vi "Update Gas desk files.vi"() -> ()   [LabVIEW 2011]
uses:
  Controls/File_Selector_Type.ctl
panel:
  out "Current file":path
  in  "Previous Choice":path
  in  "Search String":string
  in  "At Dialog Prompt Post Process":T1
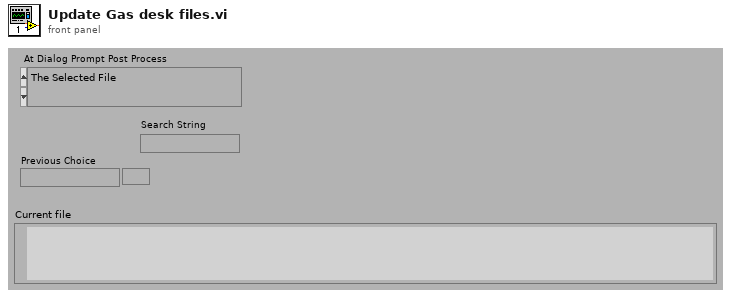
[diagram p1: front panel]
types:
  T1 = typedef "File_Selector_Type.ctl" = enum16{"The Selected File", "The Selected Folder", "Files containing the search string in the selected folder", "All files listed in selected file"}
  T2 = enum16{"To Traverse Coordinates", "To User Coordinates"}
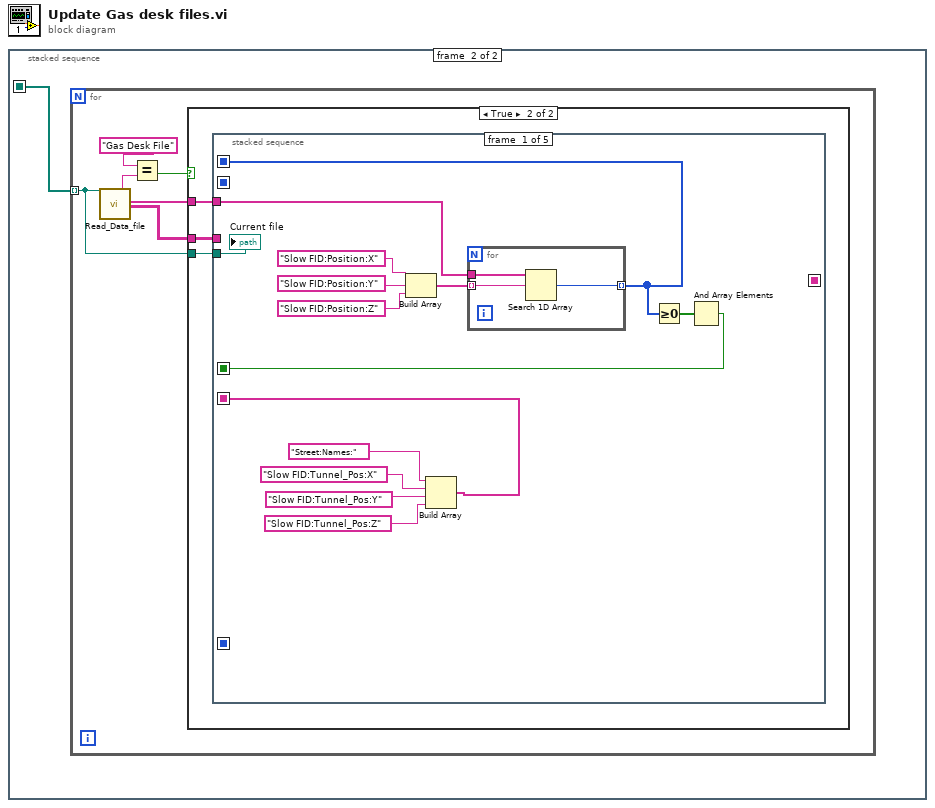
[diagram p0: block diagram]
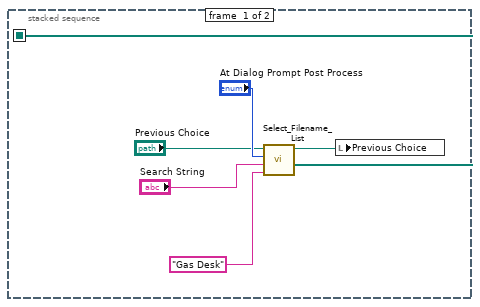
[diagram p2: hidden frame]
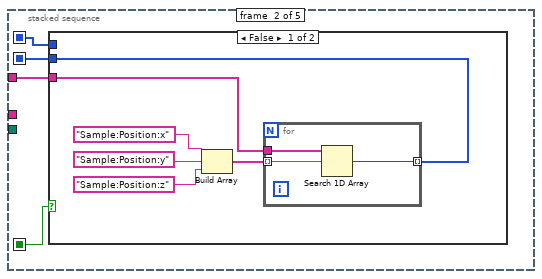
[diagram p4: hidden frame]
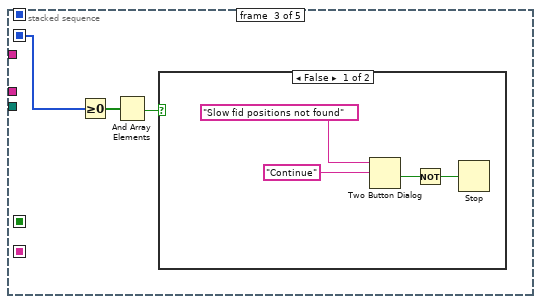
[diagram p6: hidden frame]
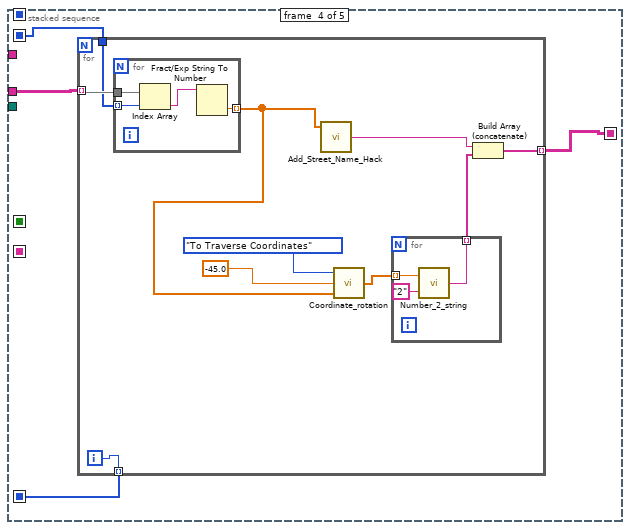
[diagram p8: hidden frame]
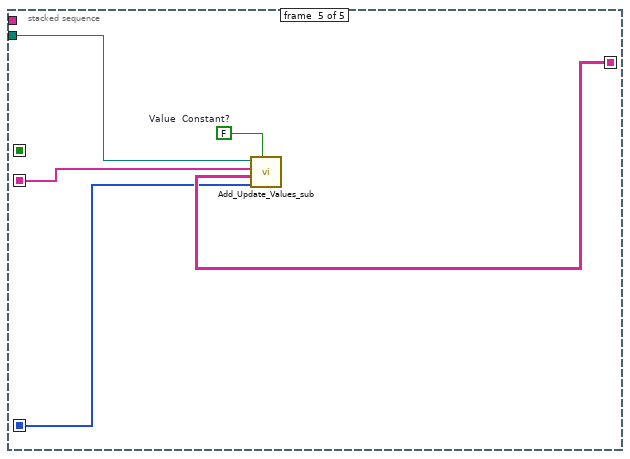
[diagram p9: hidden frame]
diagram:
  n1 = stacked-sequence {
    seq-local: [w1 _] -> [_ w7]
    frame #0 {
      n2 = call "Select_Filename_List.vi"("File Type"="Gas Desk", "Search String"="Search String", "At Dialog Prompt Post Process"="At Dialog Prompt Post Process", "Previous Choice"="Previous Choice") -> ("Selected files"=w1:path[], "Choosen path"=w4:path)  [unwired: 2 in, 1 out]
      n3 = local write "Previous Choice"(w4) -> ()
    }
    frame #1 {
      n4 = for {
        tunnel: w7 -> [w8] mode=indexing
        n5 = call "Read_Data_file.vi"("Results file"=w8) -> ("Filetype"=w13:string, "Ch names Out"=w10:string[], "Channel Values Out"=w9:string[][])  [unwired: 9 in, 7 out]
        n6 = Equal?(x="Gas Desk File", y=w13) -> (x = y?=w11:bool)
        n7 = case shown="True" w11 {
          tunnel: w10 -> [_ w16]
          tunnel: w9 -> [_ w15]
          tunnel: w8 -> [_ w14]
          frame False {
          }
          frame True {
            n8 = stacked-sequence {
              seq-local: [w20 _ _ _ _] -> [_ w34 _ _ _]
              seq-local: [w21 _ _ _ _] -> [_ _ _ _ w79]
              seq-local: [_ _ _ w57 _] -> [_ _ _ _ w78]
              seq-local: [_ _ _ w56 _] -> [_ _ _ _ w77]
              seq-local: [w18 _ _ _ _] -> [_ w36 _ _ _]
              seq-local: [_ w35 _ _ _] -> [_ _ w49 w55 _]
              tunnel: w16 -> [w26 w37 _ _ _]
              tunnel: w15 -> [_ _ _ w58 _]
              tunnel: w14 -> [w17 _ _ _ w80]
              frame #0 {
                n9 = Build Array("Slow FID:Position:X", "Slow FID:Position:Y", "Slow FID:Position:Z") -> (w27:string[])
                n10 = Build Array("Street:Names:", "Slow FID:Tunnel_Pos:X", "Slow FID:Tunnel_Pos:Y", "Slow FID:Tunnel_Pos:Z") -> (w21:string[])
                n11 = for {
                  tunnel: w27 -> [w33] mode=indexing
                  tunnel: w26 -> [w32]
                  tunnel: [w31] -> w20 mode=indexing
                  n12 = Search 1D Array(1D array=w32, element=w33) -> (index of element=w31:i32)  [unwired: 1 in]
                }
                n13 = Greater Or Equal To 0?(x=w20) -> (x >= 0?=w19:bool[])
                n14 = And Array Elements(Boolean array=w19) -> (logical AND=w18:bool)
                "Current file" <- w17
              }
              frame #1 {
                n15 = case shown="False" w36 {
                  tunnel: w37 -> [w39 _]
                  tunnel: [w38 w47] -> w35
                  tunnel: w34 -> [_ w47]
                  frame False {
                    n16 = Build Array("Sample:Position:x", "Sample:Position:y", "Sample:Position:z") -> (w40:string[])
                    n17 = for {
                      tunnel: w40 -> [w46] mode=indexing
                      tunnel: w39 -> [w45]
                      tunnel: [w44] -> w38 mode=indexing
                      n18 = Search 1D Array(1D array=w45, element=w46) -> (index of element=w44:i32)  [unwired: 1 in]
                    }
                  }
                  frame True {
                  }
                }
              }
              frame #2 {
                n19 = Greater Or Equal To 0?(x=w49) -> (x >= 0?=w50:bool[])
                n20 = And Array Elements(Boolean array=w50) -> (logical AND=w48:bool)
                n21 = case shown="False" w48 {
                  frame False {
                    n22 = Two Button Dialog(message="Slow fid positions not found", 2:"Continue" ("T button name (\"OK\")")) -> (T button?=w52:bool)  [unwired: 1 in]
                    n23 = Not(x=w52) -> (.not. x?=w51:bool)
                    n24 = Stop(stop? (T)=w51) -> ()
                  }
                  frame True {
                  }
                }
              }
              frame #3 {
                n25 = for {
                  tunnel: w58 -> [w68] mode=indexing
                  tunnel: w55 -> [w67]
                  tunnel: [w61] -> w57 mode=indexing
                  tunnel: [w60] -> w56 mode=indexing
                  i -> [w60]
                  n26 = for {
                    tunnel: w68 -> [w75]
                    tunnel: w67 -> [w74] mode=indexing
                    tunnel: [w72] -> w65 mode=indexing
                    n27 = Index Array(array=w75, index=w74) -> (element=w73:string)
                    n28 = Fract/Exp String To Number(string=w73) -> (number=w72:dbl)  [unwired: 3 in, 1 out]
                  }
                  n29 = call "Add_Street_Name_Hack.vi"("Model Input Position"=w65) -> ("Street Names"=w62:string)  [unwired: 6 in]
                  n30 = call "Coordinate_rotation.vi"("Input Position"=w65, "Coordinate rotation (deg)"=-45.0, "Mode"=T2."To Traverse Coordinates") -> ("Output Position"=w64:dbl[])
                  n31 = for {
                    tunnel: w64 -> [w71] mode=indexing
                    tunnel: [w69] -> w63 mode=indexing
                    n32 = call "Number_2_string.vi"("precision"="2", "number"=w71) -> ("String"=w69:string)
                  }
                  n33 = Build Array (concatenate)(w62, w63) -> (w61:string[])
                }
              }
              frame #4 {
                w76 = FALSE  # Value  Constant?
                n34 = call "Add_Update_Values_sub.vi"("Value  Constant?"=w76, "Selected Rows"=w77, "New Values In"=w78, "New Chs In"=w79, "Filename"=w80) -> ()  [unwired: 6 in, 1 out]
              }
            }
          }
        }
      }
    }
  }
